vi "SplitIPandPort.vi"(10 "defaultPort(10001)":u16=10001, 11 "IP:Port":string) -> (2 "Port":u16, 3 "IP":string)   [LabVIEW 2017]
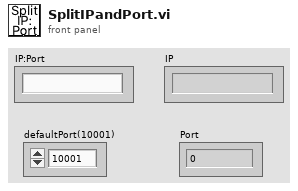
[diagram p1: front panel]
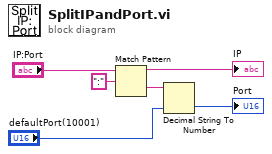
[diagram p0: block diagram]
diagram:
  n1 = Match Pattern(string="IP:Port", regular expression=":") -> (before substring=→"IP":string, after substring=w4:string)  [unwired: 1 in, 2 out]
  n2 = Decimal String To Number(string=w4, default (0L)="defaultPort(10001)") -> (number=→"Port":u16)  [unwired: 1 in, 1 out]
